vi "Write 1st Instrument.vi"(8 "error in (no error)":errorcluster, 10 "RP Instrument.lvclass":refnum<class "RP Instrument.lvclass">, 11 "Red Pitaya Digitizer in":refnum<class "Red Pitaya Digitizer.lvclass">) -> (0 "error out":errorcluster, 3 "Red Pitaya Digitizer out":refnum<class "Red Pitaya Digitizer.lvclass">)   [LabVIEW 2024, in "Red Pitaya Digitizer.lvclass"]
uses:
  Red Pitaya Digitizer.lvclass
  RP Core/RP Instrument/RP Instrument.lvclass
  Red Pitaya Digitizer.lvclass/Red Pitaya Digitizer.ctl
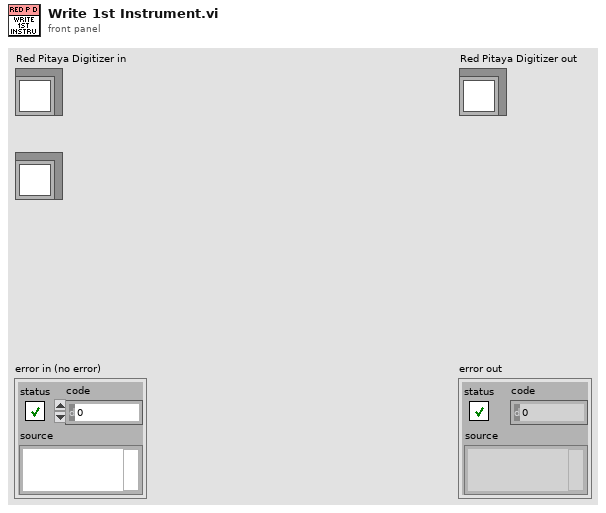
[diagram p1: front panel]
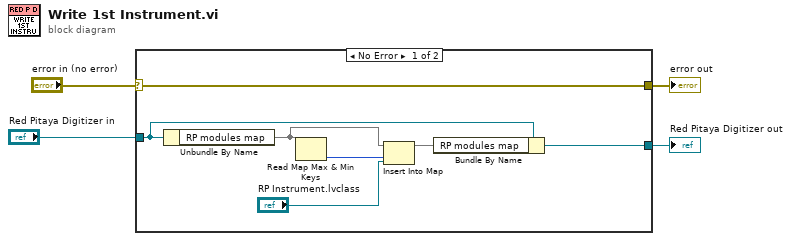
[diagram p0: block diagram]
diagram:
  n1 = case shown="No Error" "error in (no error)" {
    selector: "error in (no error)" -> [w11 w13]
    tunnel: [w11 w13] -> w3
    tunnel: [w9 w12] -> w1
    tunnel: "Red Pitaya Digitizer in" -> [w10 w12]
    frame No Error {
      n2 = Unbundle By Name(w10) -> ("RP modules map"=w8:map{i32, refnum<class "RP Instrument.lvclass">})
      n3 = Read Map Max & Min Keys(11:w8) -> (1:w7:i32)  [unwired: 1 out]
      n4 = Insert Into Map(map in=w8, key=w7, value="RP Instrument.lvclass") -> (map out=w5:map{i32, refnum<class "RP Instrument.lvclass">})  [unwired: 2 out]
      n5 = Bundle By Name(cluster=w10, "RP modules map"=w5) -> (w9:refnum<class "Red Pitaya Digitizer.lvclass">)
    }
    frame Error {
    }
  }
  "error out" <- w3
  "Red Pitaya Digitizer out" <- w1
